vi "LibXML_FirstMatchContent.vi"(8 "error in":errorcluster, 9 "rootnode (root of doc)":u32, 10 "xpathexpr":string="/ScanMaster/Devices/Device/description", 11 "doc in":u32) -> (0 "error out":errorcluster, 2 "content":string="the piezo x axis via adwin analog out", 3 "doc copy out":u32)   [LabVIEW 2019, in "Tools.lvlib"]
doc: "gets the content of the first matched node only."
uses:
  Tools.lvlib
  Error Cluster From Error Code_subroutine.vi
  <vilib>/Utility/error.llb/Trim Whitespace.vi
  LibXML.lvlib
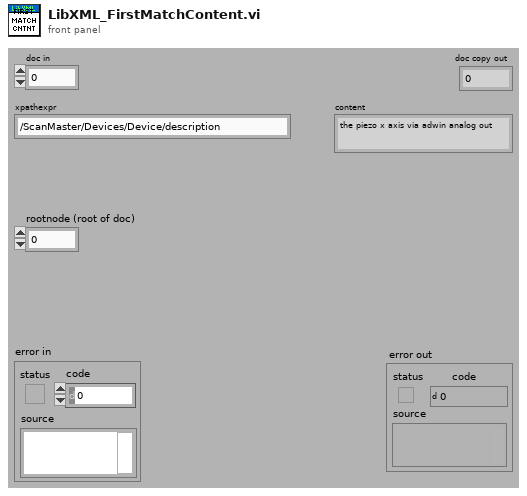
[diagram p1: front panel]
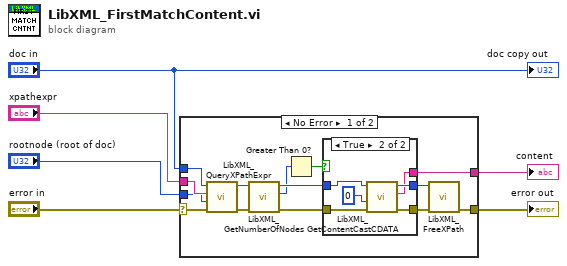
[diagram p0: block diagram]
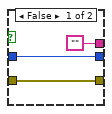
[diagram p2: hidden frame]
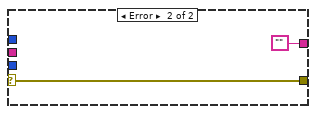
[diagram p3: hidden frame]
diagram:
  n1 = case shown="No Error" "error in" {
    selector: "error in" -> [w7 w31]
    tunnel: "xpathexpr" -> [w20 _]
    tunnel: [w18 w31] -> w5
    tunnel: "doc in" -> [w16 _]
    tunnel: [w15 ""] -> w3
    tunnel: "rootnode (root of doc)" -> [w14 _]
    frame No Error {
      n2 = call "LibXML_QueryXPathExpr.vi"("error in"=w7, "rootnode (root of doc)"=w14, "XPathExpr"=w20, "doc"=w16) -> ("error out"=w13:errorcluster, "xmlXPathObj"=w12:u32)  [unwired: 6 in]
      n3 = call "LibXML_GetNumberOfNodes.vi"("error in (no error)"=w13, "XPathObj"=w12) -> ("error out"=w11:errorcluster, "#ofNodes"=w9:i32, "XPathObj out"=w10:u32)  [unwired: 7 in]
      n4 = Greater Than 0?(x=w9) -> (x > 0?=w8:bool)
      n5 = case shown="True" w8 {
        tunnel: [w22 w29] -> w19
        tunnel: [w21 w28] -> w17
        tunnel: ["" w26] -> w15
        tunnel: w11 -> [w21 w25]
        tunnel: w10 -> [w22 w24]
        frame False {
        }
        frame True {
          n6 = call "LibXML_GetContentCastCDATA.vi"("error in"=w25, "index"=0, "xmlXPathObj"=w24) -> ("error out"=w28:errorcluster, "content"=w26:string, "xmlXPathObj out"=w29:u32)  [unwired: 6 in]
        }
      }
      n7 = call "LibXML_FreeXPath.vi"("error in"=w17, "XPathObj"=w19) -> ("error out"=w18:errorcluster)  [unwired: 9 in]
    }
    frame Error {
    }
  }
  "content" <- w3
  "error out" <- w5
  "doc copy out" <- "doc in"
